vi "Scan Page for bricks to fall.vi"(10 "Page Index":i32, 11 "Block Array":i32[][][](array[numeric])) -> (3 "Fall IDs":i32[](array[numeric]))   [LabVIEW 2023]
uses:
  <vilib>/Utility/miscctls.llb/LVMapReplaceAction.ctl
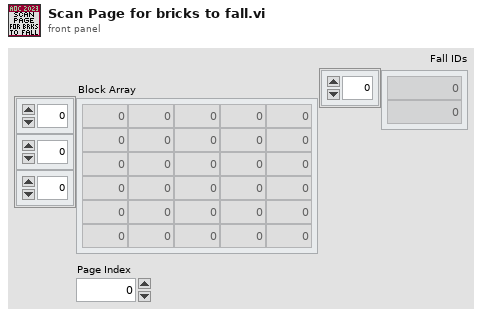
[diagram p1: front panel]
types:
  T1 = typedef "LVMapReplaceAction.ctl" = enum32{"Modify Entry only if found", "Add or Modify Entry", "Delete Entry"}
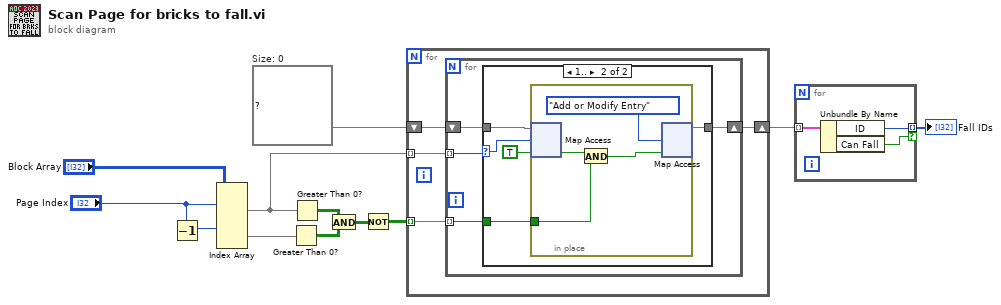
[diagram p0: block diagram]
diagram:
  w12 = map{i32, bool} {}  # Size: 0
  n1 = Decrement(x="Page Index") -> (x-1=w4:i32)
  n2 = Index Array(array="Block Array", index (dim 0) #1="Page Index", index (dim 0) #2=w4) -> (element #1=w10:i32[][], element #2=w6:i32[][])  [unwired: 4 in]
  n3 = Greater Than 0?(x=w6) -> (x > 0?=w8:bool[][])
  n4 = Greater Than 0?(x=w10) -> (x > 0?=w7:bool[][])
  n5 = And(x=w7, y=w8) -> (x .and. y?=w9:bool[][])
  n6 = Not(x=w9) -> (.not. x?=w11:bool[][])
  n7 = for {
    tunnel: w10 -> [w15] mode=indexing
    tunnel: w11 -> [w16] mode=indexing
    shift-right: [w13] -> w2
    shift-left: w12 -> [w14]
    n8 = for {
      tunnel: w16 -> [w17] mode=indexing
      tunnel: w15 -> [w20] mode=indexing
      shift-right: [w18] -> w13
      shift-left: w14 -> [w19]
      n9 = case shown="1.." w20 {
        selector: w20 -> [_ w25]
        tunnel: w19 -> [w21 w26]
        tunnel: [w21 w22] -> w18
        tunnel: w17 -> [_ w23]
        frame ..0 {
        }
        frame 1.. {
          n10 = in-place {
            in-place-border: w23 -> [w28]
            n11 = in-place-map #1(w26, w25, TRUE ("Can Fall")) -> (w29:bool)  [unwired: 1 out]
            n12 = And(x=w29, y=w28) -> (x .and. y?=w27:bool)
            n13 = in-place-map #1(w27, LVMapReplaceAction."Add or Modify Entry" ("action")) -> (w22:map{i32, bool})  [unwired: 2 out]
          }
        }
      }
    }
  }
  n14 = for {
    tunnel: w2 -> [w33] mode=indexing
    tunnel: [w32] -> w1 mode=indexing if=w31
    n15 = Unbundle By Name(w33) -> ("ID"=w32:i32, "Can Fall"=w31:bool)
  }
  "Fall IDs" <- w1
